vi "Load Session.vi"(8 "error in (no error)":errorcluster, 10 "Hashed ID":string, 11 "Session in":refnum<class "Session.lvclass">) -> (0 "error out":errorcluster, 3 "Session out":refnum<class "Session.lvclass">)   [LabVIEW 2020, in "HTTP Server.lvlib" / "Session.lvclass"]
uses:
  Session.lvclass
  Session.lvclass/Session.ctl
  <vilib>/Utility/error.llb/Error Cluster From Error Code.vi
  <vilib>/ErrorRing/Error Ring.xnode
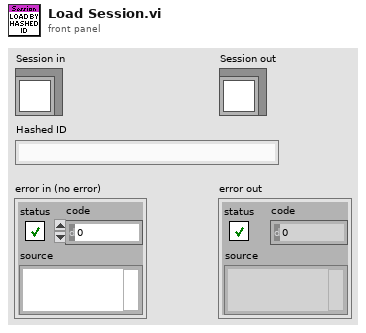
[diagram p1: front panel]
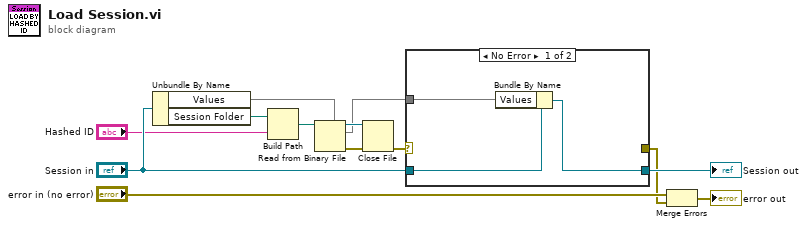
[diagram p0: block diagram]
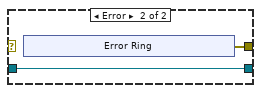
[diagram p2: hidden frame]
diagram:
  n1 = Unbundle By Name("Session in") -> ("Values"=w6:map{string, string}, "Session Folder"=w13:path)
  n2 = Build Path(base path=w13, name or relative path="Hashed ID") -> (appended path=w7:path)
  n3 = Read from Binary File(5:w6, 11:w7) -> (0:w9:errorcluster, 2:w8:map{string, string}, 3:w10:refnum<file>)  [unwired: 4 in, 1 out]
  n4 = Close File(refnum=w10, error in=w9) -> (error out=w5:errorcluster)  [unwired: 1 out]
  n5 = case shown="No Error" w5 {
    tunnel: "Session in" -> [w16 w18]
    tunnel: [w15 w18] -> w11
    tunnel: w8 -> [w14 _]
    tunnel: [_ w17] -> w3
    frame No Error {
      n6 = Bundle By Name(cluster=w16, "Values"=w14) -> (w15:refnum<class "Session.lvclass">)
    }
    frame Error {
      n7 = xnode "Error Ring"() -> ("error out"=w17:errorcluster)
    }
  }
  "Session out" <- w11
  n8 = Merge Errors("error in (no error)", w3) -> (→"error out":errorcluster)
